vi "deserializeMissionArray.vi"(8 "Error In":errorcluster, 11 "Serialized Mission Array":string) -> (0 "Error Out":errorcluster, 3 "Mission Object Array":refnum<class "GenericMission.lvclass">[](array[class]))   [LabVIEW 2011]
uses:
  GenericMission/GenericMission.lvclass
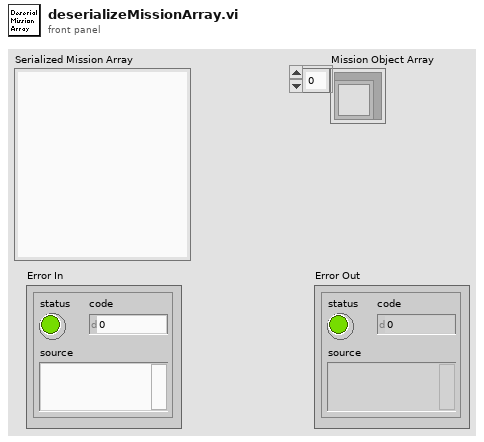
[diagram p1: front panel]
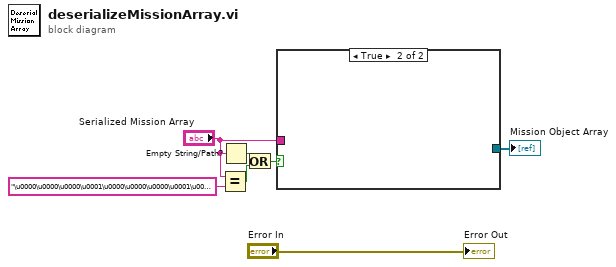
[diagram p0: block diagram]
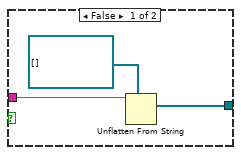
[diagram p2: hidden frame]
diagram:
  n1 = Equal?(x="Serialized Mission Array", y="\u0000\u0000\u0000\u0001\u0000\u0000\u0000\u0001\u0018\u0016GenericMission.lvclass\u0000\u0000\u0000\u0000\u0000\u0000\u0000\u0000\u0000\u0000\u0000\u0000" ("x")) -> (x = y?=w1:bool)
  n2 = Empty String/Path?(string/path="Serialized Mission Array") -> (empty?=w7:bool)
  n3 = Or(x=w7, y=w1) -> (x .or. y?=w2:bool)
  n4 = case shown="True" w2 {
    tunnel: [w9 _] -> w6
    tunnel: "Serialized Mission Array" -> [w10 _]
    frame False {
      n5 = Unflatten From String(type=refnum<class "GenericMission.lvclass">[] [] ("Mission Object Array"), binary string=w10) -> (value=w9:refnum<class "GenericMission.lvclass">[])  [unwired: 3 in, 2 out]
    }
    frame True {
    }
  }
  "Mission Object Array" <- w6
  "Error Out" <- "Error In"
